vi "room put all.vi"(8 "error in (no error)":errorcluster, 9 "R3?":bool, 10 "side?":bool, 11 "main.ctl":T1) -> (0 "error out":errorcluster, 3 "main.ctl 2":T1)   [LabVIEW 2019]
uses:
  main data.ctl
  vision/vision_board_ctl.ctl
  block box.ctl
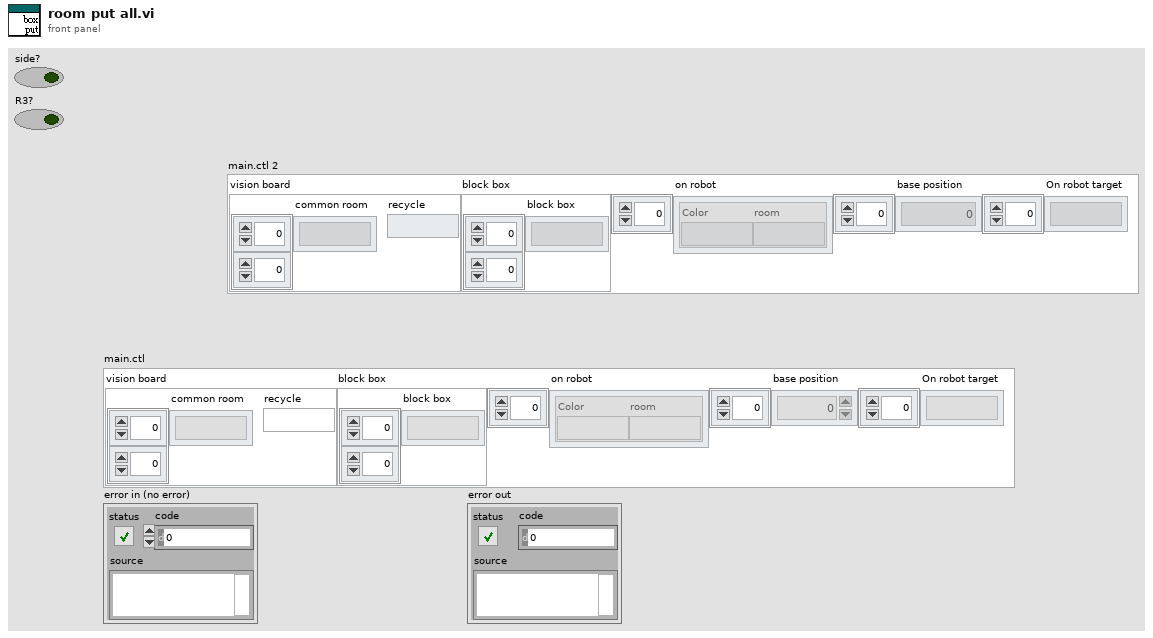
[diagram p1: front panel]
types:
  T1 = typedef "main data.ctl" = cluster{"vision board":T2, "block box":T3, "on robot ":cluster{"Color":string, "room":string}[], "base position":dbl[], "On robot target":string[]}
  T2 = typedef "vision_board_ctl.ctl" = cluster{"common room":string[][], "recycle":string}
  T3 = typedef "block box.ctl" = cluster{"block box":string[][]}
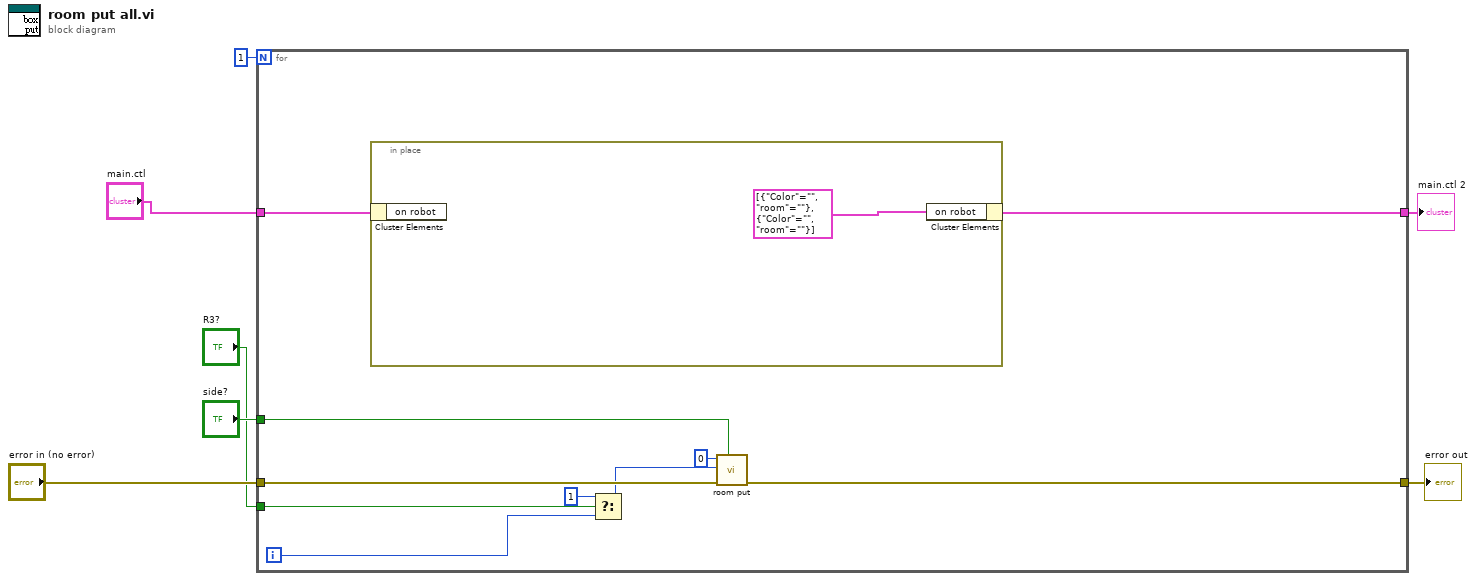
[diagram p0: block diagram]
diagram:
  n1 = for {
    N: 1 -> [_]
    tunnel: "main.ctl" -> [w17]
    tunnel: "error in (no error)" -> [w16]
    tunnel: [w15] -> w5
    tunnel: [w14] -> w4
    tunnel: "side?" -> [w13]
    tunnel: "R3?" -> [w9]
    i -> [w11]
    n2 = in-place {
      n3 = in-place-cluster #1(w17) -> ()  [unwired: 1 out]
      n4 = in-place-cluster #1("on robot"=cluster{"Color":string, "room":string}[] [{"Color"="", "room"=""}, {"Color"="", "room"=""}]) -> (w14:T1)
    }
    n5 = Select(t=1, s=w9, f=w11) -> (s? t:f=w12:i32)
    n6 = call "room put.vi"("side?"=w13, "error in (no error)"=w16, "register address"=w12, "put layer"=0) -> ("error out"=w15:errorcluster)  [unwired: 6 in, 1 out]
  }
  "error out" <- w5
  "main.ctl 2" <- w4
